vi "SetClimbSpeed.vi"(10 "Climb Speed":dbl, 11 "Climber in":refnum<class "Climber.lvclass">) -> (3 "Climber out":refnum<class "Climber.lvclass">)   [LabVIEW 2016, in "Climber.lvclass"]
uses:
  Climber.lvclass
  Climber.lvclass/Climber.ctl
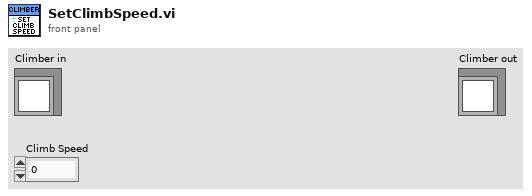
[diagram p1: front panel]
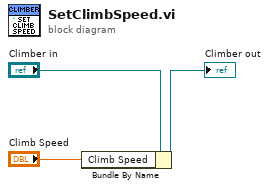
[diagram p0: block diagram]
diagram:
  n1 = Bundle By Name(cluster="Climber in", "Climb Speed"="Climb Speed") -> (→"Climber out":refnum<class "Climber.lvclass">)
